vi "Load Past Report Info.vi"(8 "error in (no error)":errorcluster, 11 "Report Path":path) -> (0 "error out":errorcluster, 1 "Valid Report":bool, 2 "SubTests Select Data.Completed SubTests Array":T3[](array[typedef]), 3 "APU Select":T2, 4 "Test Information":T1)   [LabVIEW 2018, in "File IO.lvlib"]
uses:
  File IO.lvlib
  Controller (Host)/Public Controls/SubTest Data.ctl
  Controller (Host)/Public Controls/APU Select.ctl
  Controller (Host)/Public Controls/Test Information.ctl
  <vilib>/addons/_office/excel.llb/Excel Get Data ([str]).vi
  <vilib>/Utility/NIReport.llb/NI_report.lvclass
  <vilib>/Utility/NIReport.llb/Excel/NI_Excel.lvclass
  <vilib>/addons/_office/NI_ReportGenerationToolkit.lvlib
  Controller (Host)/Controller (Host).lvlib
panel:
  # "Test Information:"
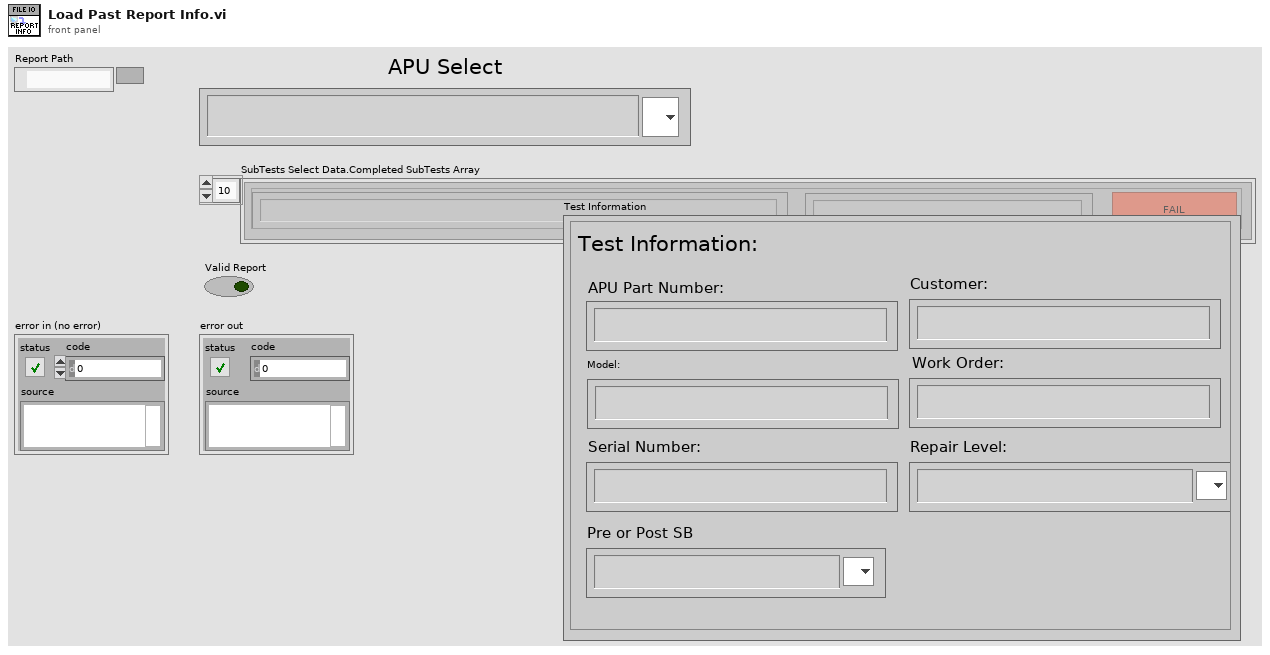
[diagram p1: front panel]
types:
  T1 = typedef "Controller (Host).lvlib/Test Information.ctl" = cluster{"APU Part Number:":string, "Model:":string, "Serial Number:":string, "Customer:":string, "Work Order:":string, "Repair Level:":string, "Pre or Post SB":string}
  T2 = typedef "Controller (Host).lvlib/APU Select.ctl" = string
  T3 = typedef "Controller (Host).lvlib/SubTest Data.ctl" = cluster{"SubTest":string, "End Time":string, "Fail/Pass":bool, "Cover Data":bool}
  T4 = enum16{"maximized", "minimized", "normal", "no change"}
  T5 = enum16{"Standard Report", "HTML", "Word", "Excel"}
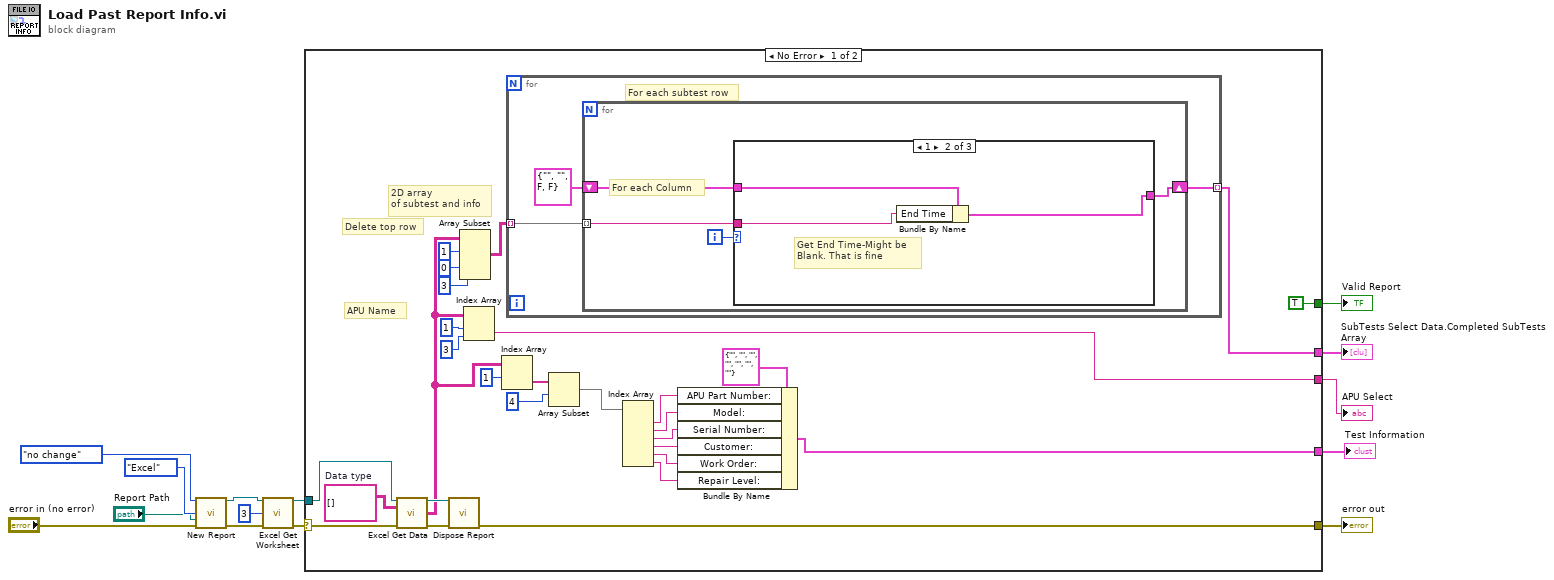
[diagram p0: block diagram]
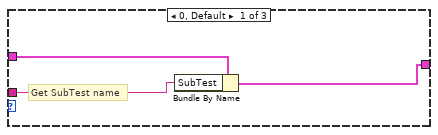
[diagram p2: hidden frame]
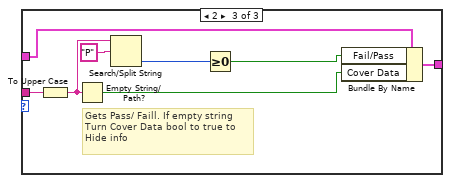
[diagram p3: hidden frame]
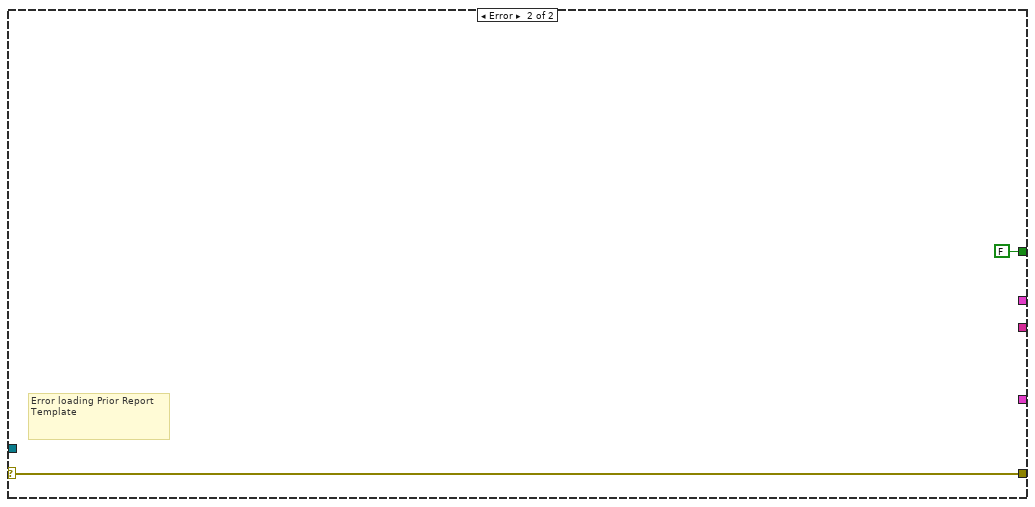
[diagram p4: hidden frame]
diagram:
  n1 = call <vilib>:"New Report.vi"("window state (normal)"=T4."no change", "report type"=T5."Excel", "template (empty)"="Report Path", "error in (no error)"="error in (no error)") -> ("report out"=w7:refnum<class "NI_report.lvclass">, "error out"=w8:errorcluster)  [unwired: 10 in]
  n2 = call <vilib>:"Excel Get Worksheet.vi"("report in"=w7, "worksheet index (0)"=3, "error in (no error)"=w8) -> ("report out"=w4:refnum<class "NI_report.lvclass">, "error out"=w5:errorcluster)  [unwired: 11 in]
  n3 = case shown="No Error" w5 {
    selector: w5 -> [w42 w64]
    tunnel: [w37 w64] -> w14
    tunnel: [TRUE ("Valid Report") FALSE ("Valid Report")] -> w13
    tunnel: w4 -> [w40 _]
    tunnel: [w33 _] -> w3
    tunnel: [w32 _] -> w2
    tunnel: [w20 _] -> w1
    frame No Error {
      w41 = string[][] []  # Data type
      # "APU Name"
      # "Delete top row"
      # "2D array\nof subtest and info"
      n4 = call-poly <vilib>:"Excel Get Data.vi"("report in"=w40, "data type"=w41, "error in (no error)"=w42) -> ("report out"=w36:refnum<class "NI_report.lvclass">, "data"=w19:string[][], "error out"=w38:errorcluster)  [unwired: 10 in]
      n5 = call-dynamic "Dispose Report.vi"("report in"=w36, "error in (no error)"=w38) -> ("error out"=w37:errorcluster)  [unwired: 13 in]
      n6 = Array Subset(array=w19, index (row)=1 ("index"), index (col)=0 ("index"), length (col)=3 ("length")) -> (w18:string[][])  [unwired: 1 in]
      n7 = Index Array(array=w19, index (row)=1, index (col)=3 ("disabled index (col)")) -> (element=w33:string)
      n8 = Index Array(array=w19, index (row)=1) -> (element=w29:string[])  [unwired: 1 in]
      n9 = for {
        tunnel: w18 -> [w45] mode=indexing
        tunnel: [w43] -> w32 mode=indexing
        # "For each subtest row"
        n10 = for {
          tunnel: w45 -> [w47] mode=indexing
          shift-right: [w48] -> w43
          shift-left: T3 {"SubTest"="", "End Time"="", "Fail/Pass"=FALSE, "Cover Data"=FALSE} ("Completed SubTest Data") -> [w46]
          i -> [w49]
          # "For each Column"
          n11 = case shown="1" w49 {
            tunnel: w46 -> [w52 w53 w62]
            tunnel: [w51 w55 w63] -> w48
            tunnel: w47 -> [w50 w54 w61]
            frame 0, Default {
              # "Get SubTest name"
              n12 = Bundle By Name(cluster=w52, "SubTest"=w50) -> (w51:T3)
            }
            frame 1 {
              # "Get End Time-Might be\nBlank. That is fine"
              n13 = Bundle By Name(cluster=w53, "End Time"=w54) -> (w55:T3)
            }
            frame 2 {
              # "Gets Pass/ Faill. If empty string\nTurn Cover Data bool to true to \nHide info"
              n14 = To Upper Case(1:w61) -> (0:w59:string)
              n15 = Empty String/Path?(string/path=w59) -> (empty?=w60:bool)
              n16 = Search/Split String(string=w59, search string/char (-)="P") -> (offset of match=w57:i32)  [unwired: 1 in, 2 out]
              n17 = Greater Or Equal To 0?(x=w57) -> (x >= 0?=w56:bool)
              n18 = Bundle By Name(cluster=w62, "Fail/Pass"=w56, "Cover Data"=w60) -> (w63:T3)
            }
          }
        }
      }
      n19 = Array Subset(array=w29, index=4) -> (w27:string[])  [unwired: 1 in]
      n20 = Index Array(array=w27) -> (element #1=w26:string, element #2=w25:string, element #3=w24:string, element #4=w23:string, element #5=w22:string, element #6=w21:string)  [unwired: 6 in]
      n21 = Bundle By Name(cluster=T1 {"APU Part Number:"="", "Model:"="", "Serial Number:"="", "Customer:"="", "Work Order:"="", "Repair Level:"="", "Pre or Post SB"=""} ("Test Information"), "APU Part Number:"=w26, "Model:"=w25, "Serial Number:"=w24, "Customer:"=w23, "Work Order:"=w22, "Repair Level:"=w21) -> (w20:T1)
    }
    frame Error {
      # "Error loading Prior Report \nTemplate"
    }
  }
  "error out" <- w14
  "Valid Report" <- w13
  "SubTests Select Data.Completed SubTests Array" <- w2
  "APU Select" <- w3
  "Test Information" <- w1
